vi "Smart Mech Drive.vi"(4 "navX Device":T7={"Interface"={"Protocol"=enum."SPI", "Update Rate (4Hz-100Hz)"=50, "navX Open TypeDef"=variant(cluster{"SPI Bus":enum16{"SPI On-Board, CS0", "SPI On-Board, CS1", "SPI On-Board, CS2", "SPI On-Board, CS3", "SPI MXP", "Invalid"}, "Clock Rate (Hz)":dbl} {"SPI Bus"=enum."SPI MXP", "Clock Rate (Hz)"=2000000.0})}, "Notify Packet"=refnum, "Loop VI Refnum"=refnum, "Ready to Close Occurrence Refnum"=refnum} {"Interface"."Update Rate (4Hz-100Hz)" min=4 max=60 step=1}, 5 "rotation lock":bool, 6 "align":bool, 7 "set_angle":dbl, 10 "motor values":dbl[](array[numeric])=[0.0, 0.0, 0.0, 0.0], 11 "motor references":T1[](array[typedef])=[{"DeviceStatus"={"status"=FALSE, "code"=0, "source"=""}, "Type"=enum."CAN", "PWM"={"PWM Channel"=enum."PWM 1", "DeadBand"={"Name"="", "maxPositivePwm"=0, "minPositivePwm"=0, "centerPwm"=0, "maxNegativePwm"=0, "minNegativePwm"=0, "angularRange"=0}}, "CAN"={"Device Number"=2, "SetOutput VI Ref"=variant(refnum<vi> refnum), "GetOutput VI Ref"=variant(refnum<vi> refnum), "Enable VI Ref"=variant(refnum<vi> refnum), "Disable VI Ref"=variant(refnum<vi> refnum), "Data"=variant(cluster{"Library":path, "handle":u64, "Control Mode":u16, "UsageFrame":u32, "RefNumName":string, "arbID":u32} {"Library"=path "libCTRE_PhoenixCCI.so", "handle"=3032512360, "Control Mode"=0, "UsageFrame"=0, "RefNumName"="drive_fl", "arbID"=33816578})}, "Invert"=TRUE, "DIO PWM"={"PWM \"Enable\" Channel"=enum."Invalid", "DIOChannel"=enum."Invalid", "PWM Rate"=0.0}}, {"DeviceStatus"={"status"=FALSE, "code"=0, "source"=""}, "Type"=enum."CAN", "PWM"={"PWM Channel"=enum."PWM 1", "DeadBand"={"Name"="", "maxPositivePwm"=0, "minPositivePwm"=0, "centerPwm"=0, "maxNegativePwm"=0, "minNegativePwm"=0, "angularRange"=0}}, "CAN"={"Device Number"=4, "SetOutput VI Ref"=variant(refnum<vi> refnum), "GetOutput VI Ref"=variant(refnum<vi> refnum), "Enable VI Ref"=variant(refnum<vi> refnum), "Disable VI Ref"=variant(refnum<vi> refnum), "Data"=variant(cluster{"Library":path, "handle":u64, "Control Mode":u16, "UsageFrame":u32, "RefNumName":string, "arbID":u32} {"Library"=path "libCTRE_PhoenixCCI.so", "handle"=2990105016, "Control Mode"=0, "UsageFrame"=0, "RefNumName"="drive_fr", "arbID"=33816580})}, "Invert"=TRUE, "DIO PWM"={"PWM \"Enable\" Channel"=enum."Invalid", "DIOChannel"=enum."Invalid", "PWM Rate"=0.0}}, {"DeviceStatus"={"status"=FALSE, "code"=0, "source"=""}, "Type"=enum."CAN", "PWM"={"PWM Channel"=enum."PWM 1", "DeadBand"={"Name"="", "maxPositivePwm"=0, "minPositivePwm"=0, "centerPwm"=0, "maxNegativePwm"=0, "minNegativePwm"=0, "angularRange"=0}}, "CAN"={"Device Number"=3, "SetOutput VI Ref"=variant(refnum<vi> refnum), "GetOutput VI Ref"=variant(refnum<vi> refnum), "Enable VI Ref"=variant(refnum<vi> refnum), "Disable VI Ref"=variant(refnum<vi> refnum), "Data"=variant(cluster{"Library":path, "handle":u64, "Control Mode":u16, "UsageFrame":u32, "RefNumName":string, "arbID":u32} {"Library"=path "libCTRE_PhoenixCCI.so", "handle"=3032511496, "Control Mode"=0, "UsageFrame"=0, "RefNumName"="drive_rl", "arbID"=33816579})}, "Invert"=TRUE, "DIO PWM"={"PWM \"Enable\" Channel"=enum."Invalid", "DIOChannel"=enum."Invalid", "PWM Rate"=0.0}}, {"DeviceStatus"={"status"=FALSE, "code"=0, "source"=""}, "Type"=enum."CAN", "PWM"={"PWM Channel"=enum."PWM 1", "DeadBand"={"Name"="", "maxPositivePwm"=0, "minPositivePwm"=0, "centerPwm"=0, "maxNegativePwm"=0, "minNegativePwm"=0, "angularRange"=0}}, "CAN"={"Device Number"=1, "SetOutput VI Ref"=variant(refnum<vi> refnum), "GetOutput VI Ref"=variant(refnum<vi> refnum), "Enable VI Ref"=variant(refnum<vi> refnum), "Disable VI Ref"=variant(refnum<vi> refnum), "Data"=variant(cluster{"Library":path, "handle":u64, "Control Mode":u16, "UsageFrame":u32, "RefNumName":string, "arbID":u32} {"Library"=path "libCTRE_PhoenixCCI.so", "handle"=3006273360, "Control Mode"=0, "UsageFrame"=0, "RefNumName"="drive_rr", "arbID"=33816577})}, "Invert"=FALSE, "DIO PWM"={"PWM \"Enable\" Channel"=enum."Invalid", "DIOChannel"=enum."Invalid", "PWM Rate"=0.0}}]) -> (2 "new motor values":dbl[](array[numeric]), 3 "motor references":T1[](array[typedef]))   [LabVIEW 2018]
uses:
  FIRST-3958-Controls-Library/NavX/navX Library v2/TypeDefs/Z900_navX_DeviceTypeDef.ctl
  FIRST-3958-Controls-Library/NavX/navX Library v2/TypeDefs/Z900_navX_ProtocolTypeDef.ctl
  FIRST-3958-Controls-Library/NavX/navX Library v2/TypeDefs/Z900_navX_NotifyPacketTypeDef.ctl
  FIRST-3958-Controls-Library/NavX/navX Library v2/TypeDefs/Z900_navX_ActionTypeDef.ctl
  <vilib>/Rock Robotics/WPI/MotorControl/WPI_MotorControlDeviceRef.ctl
  <vilib>/Rock Robotics/WPI/MotorControl/WPI_MotorControlType.ctl
  <vilib>/Rock Robotics/SystemInterfaces/DIO/FPGA_DIOPWMChannel.ctl
  <vilib>/Rock Robotics/WPI/PWM/WPI_PWMDeadband.ctl
  <vilib>/Rock Robotics/SystemInterfaces/DIO/FPGA_DIOChannel.ctl
  <vilib>/addons/control/pid/pid.llb/PID (DBL).vi
  Robot Global Data.vi
  <vilib>/addons/control/pid/NI_PID_pid.lvlib
  FIRST-3958-Controls-Library/NavX/navX Library v2/navX Library v2.lvlib
panel:
  in  "PID gains far":T6={"proportional gain (Kc)"=1.0, "integral time (Ti, min)"=0.01, "derivative time (Td, min)"=0.0} {"derivative time (Td, min)" format="%.3f"; "integral time (Ti, min)" format="%.3f"; "proportional gain (Kc)" format="%.3f"}
  in  "PID gains":T6={"proportional gain (Kc)"=1.0, "integral time (Ti, min)"=0.01, "derivative time (Td, min)"=0.0} {"derivative time (Td, min)" format="%.3f"; "integral time (Ti, min)" format="%.3f"; "proportional gain (Kc)" format="%.3f"}
  out "Distance (ft)":dbl=nan
  in  "threshold":dbl
  in  "P":dbl=1.4
  in  "Angle PID":T6={"proportional gain (Kc)"=5.0, "integral time (Ti, min)"=0.0, "derivative time (Td, min)"=0.0} {"derivative time (Td, min)" format="%.3f"; "integral time (Ti, min)" format="%.3f"; "proportional gain (Kc)" format="%.3f"}
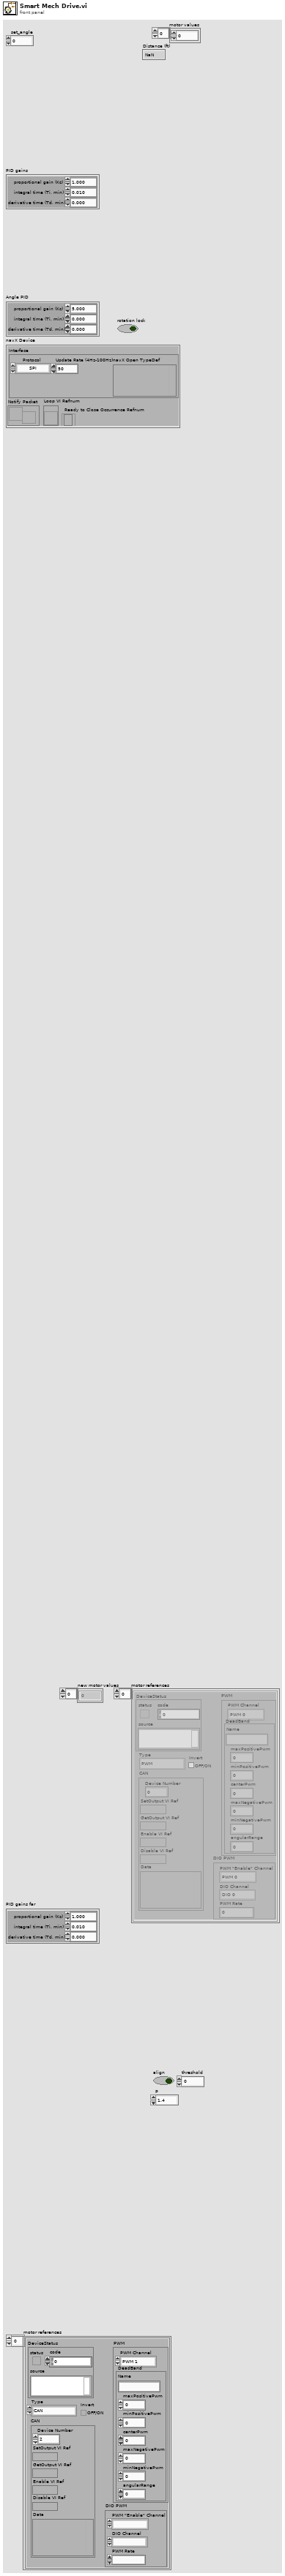
[diagram p1: front panel]
types:
  T1 = typedef "WPI_MotorControlDeviceRef.ctl" = cluster{"DeviceStatus":errorcluster, "Type":T2, "PWM":cluster{"PWM Channel":T3, "DeadBand":T4}, "CAN":cluster{"Device Number":u8, "SetOutput VI Ref":variant, "GetOutput VI Ref":variant, "Enable VI Ref":variant, "Disable VI Ref":variant, "Data":variant}, "Invert":bool, "DIO PWM":cluster{"PWM \"Enable\" Channel":T3, "DIOChannel":T5, "PWM Rate":dbl}}
  T2 = typedef "WPI_MotorControlType.ctl" = enum16{"PWM", "CAN", "DIO PWM"}
  T3 = typedef "FPGA_DIOPWMChannel.ctl" = enum8{"PWM 0", "PWM 1", "PWM 2", "PWM 3", "PWM 4", "PWM 5", "PWM 6", "PWM 7", "PWM 8", "PWM 9", "PWM MXP 0", "PWM MXP 1", "PWM MXP 2", "PWM MXP 3", "PWM MXP 4", "PWM MXP 5", "PWM MXP 6", "PWM MXP 7", "PWM MXP 8", "PWM MXP 9", "Invalid"}
  T4 = typedef "WPI_PWMDeadband.ctl" = cluster{"Name":string, "maxPositivePwm":i32, "minPositivePwm":i32, "centerPwm":i32, "maxNegativePwm":i32, "minNegativePwm":i32, "angularRange":u16}
  T5 = typedef "FPGA_DIOChannel.ctl" = enum8{"DIO 0", "DIO 1", "DIO 2", "DIO 3", "DIO 4", "DIO 5", "DIO 6", "DIO 7", "DIO 8", "DIO 9", "DIO MXP 0", "DIO MXP 1", "DIO MXP 2", "DIO MXP 3", "DIO MXP 4", "DIO MXP 5", "DIO MXP 6", "DIO MXP 7", "DIO MXP 8", "DIO MXP 9", "DIO MXP 10", "DIO MXP 11", "DIO MXP 12", "DIO MXP 13", "DIO MXP 14", "DIO MXP 15", "SPI Port CS1", "SPI Port CS2", "SPI Port CS3", "SPI Port MISO", "SPI Port MOSI", "Invalid"}
  T6 = cluster{"proportional gain (Kc)":dbl, "integral time (Ti, min)":dbl, "derivative time (Td, min)":dbl}
  T7 = typedef "navX Library v2.lvlib/Z900_navX_DeviceTypeDef.ctl" = cluster{"Interface":cluster{"Protocol":T8, "Update Rate (4Hz-100Hz)":u8, "navX Open TypeDef":variant}, "Notify Packet":refnum<notifier>, "Loop VI Refnum":refnum<vi>, "Ready to Close Occurrence Refnum":refnum<k4>}
  T8 = typedef "navX Library v2.lvlib/Z900_navX_ProtocolTypeDef.ctl" = enum16{"SERIAL", "I2C", "SPI"}
  T9 = cluster{"Yaw":dbl, "Roll":dbl, "Pitch":dbl, "Heading":dbl, "Fused Heading":dbl}
  T10 = cluster{"Distance (ft)":dbl, "Score":dbl, "Normalized":cluster{"Center":cluster{dbl, dbl}, "Rectangle":cluster{"Numeric":dbl, "Numeric 2":dbl, "Numeric 3":dbl, "Numeric 5":dbl}}, "Pixels":cluster{"Center":cluster{dbl, dbl}, "Rectangle":cluster{"Numeric":dbl, "Numeric 2":dbl, "Numeric 3":dbl, "Numeric 5":dbl}}}
  T11 = cluster{"Center":cluster{dbl, dbl}, "Rectangle":cluster{"Numeric":dbl, "Numeric 2":dbl, "Numeric 3":dbl, "Numeric 5":dbl}}
  T12 = cluster{"Numeric":dbl, "Numeric 2":dbl, "Numeric 3":dbl, "Numeric 5":dbl}
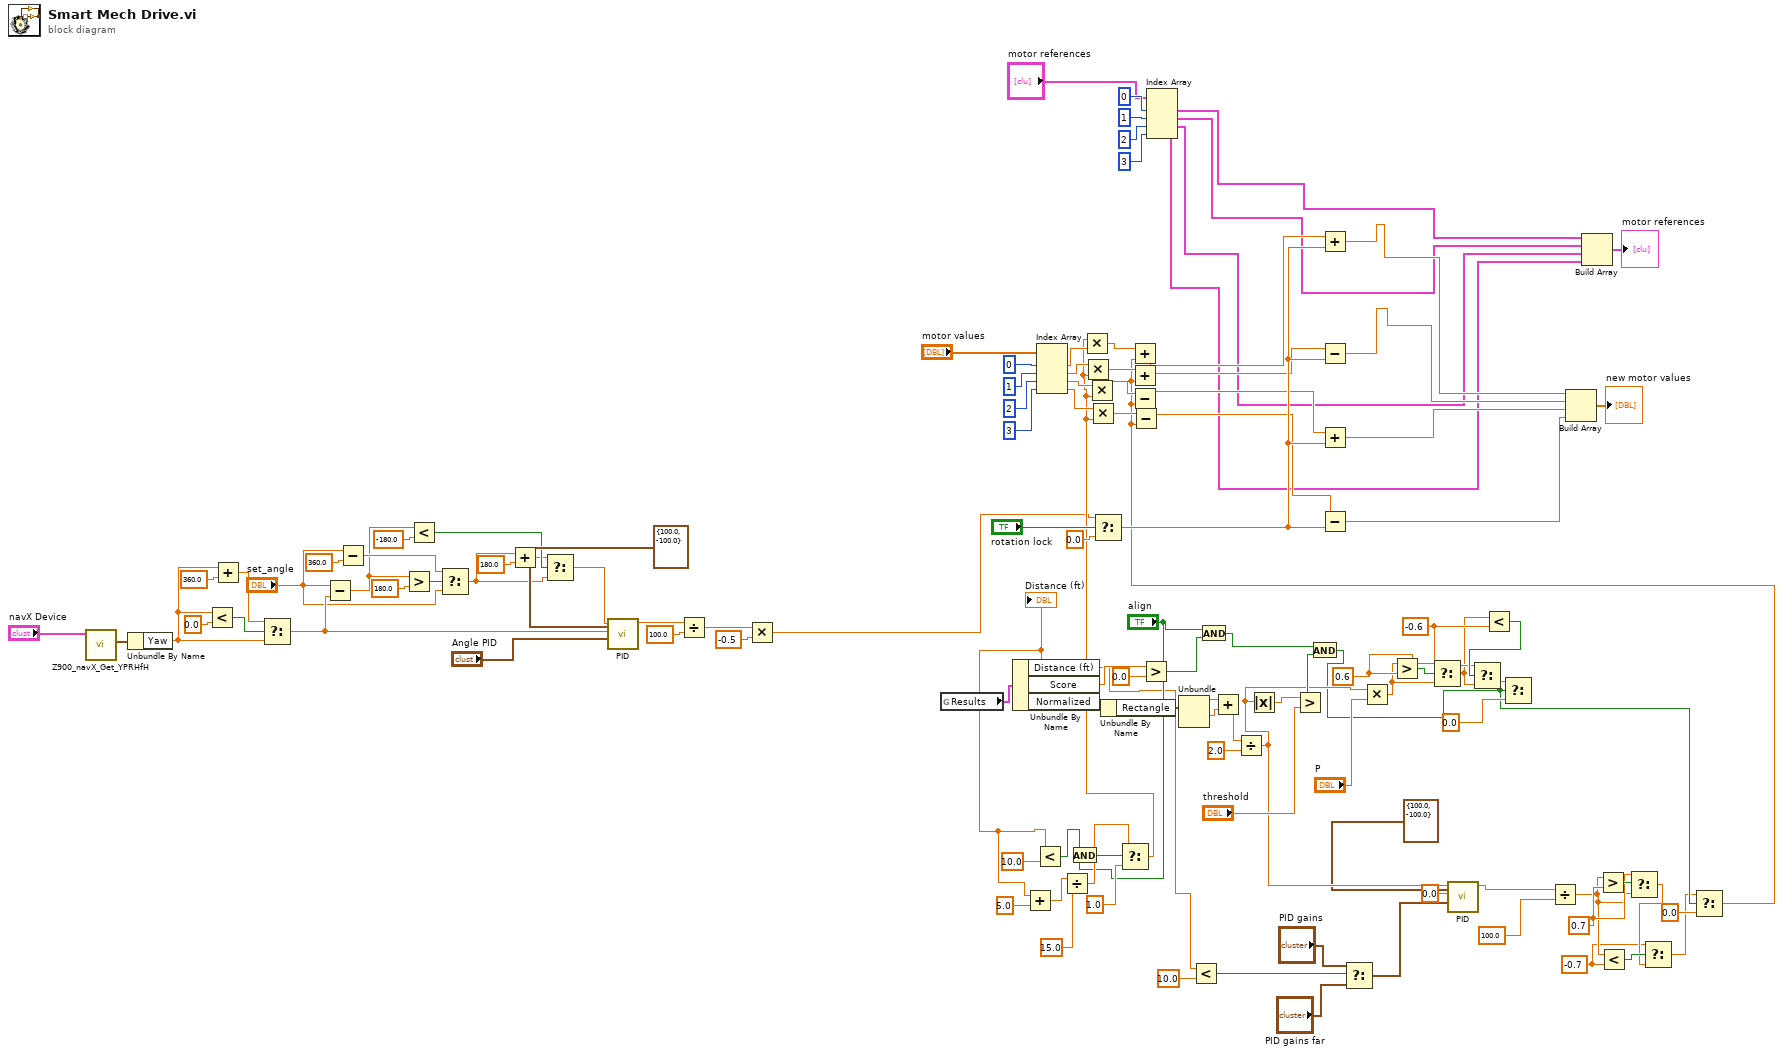
[diagram p0: block diagram]
diagram:
  w30 = -0.7 ("y")
  w34 = 0.7 ("y")
  w82 = -0.6 ("y")
  w84 = 0.6 ("y")
  n1 = call "Z900_navX_Get_YPRHfH.vi"("navX Device"="navX Device") -> ("YRPHfH"=w58:T9)  [unwired: 7 in, 3 out]
  n2 = Unbundle By Name(w58) -> ("Yaw"=w14:dbl)
  n3 = Less?(x=w14, y=0.0) -> (x < y?=w17:bool)
  n4 = Add(x=w14, y=360.0) -> (x+y=w15:dbl)
  n5 = Select(t=w15, s=w17, f=w14) -> (s? t:f=w13:dbl)
  n6 = Subtract(x="set_angle", y=w13) -> (x-y=w6:dbl)
  n7 = Subtract(x="set_angle", y=360.0) -> (x-y=w10:dbl)
  n8 = Greater?(x=w6, y=180.0) -> (0:w11:bool)
  n9 = Less?(x=w6, y=-180.0) -> (x < y?=w5:bool)
  n10 = Select(t=w10, s=w11, f="set_angle") -> (s? t:f=w4:dbl)
  n11 = Add(x=w4, y=180.0) -> (x+y=w3:dbl)
  n12 = Select(t=w3, s=w5, f=w4) -> (s? t:f=w1:dbl)
  n13 = call-poly <vilib>:"PID.vi"("output range"=cluster{"output high":dbl, "output low":dbl} {"output high"=100.0, "output low"=-100.0}, "PID gains"="Angle PID", "process variable"=w13, "setpoint"=w1) -> ("output"=w55:dbl)  [unwired: 6 in, 1 out]
  n14 = Divide(x=w55, y=100.0) -> (x/y=w53:dbl)
  n15 = Multiply(x=w53, y=-0.5) -> (x*y=w51:dbl)
  n16 = global read "Robot Global Data.vi" "Results"() -> (w105:T10)
  n17 = Unbundle By Name(w105) -> ("Distance (ft)"=w38:dbl, "Score"=w103:dbl, "Normalized"=w104:T11)
  "Distance (ft)" <- w38
  n18 = Add(x=w38, y=5.0) -> (x+y=w69:dbl)
  n19 = Less?(x=w38, y=10.0) -> (x < y?=w71:bool)
  n20 = Index Array(array="motor values", index #1=0 ("index"), index #2=1 ("index"), index #3=2 ("index"), index #4=3 ("index")) -> (element #1=w94:dbl, element #2=w108:dbl, element #3=w107:dbl, element #4=w106:dbl)
  n21 = Divide(x=w69, y=15.0) -> (x/y=w66:dbl)
  n22 = And(x=w71, y="align") -> (x .and. y?=w65:bool)
  n23 = Select(t=w51, s="rotation lock", f=0.0) -> (s? t:f=w110:dbl)
  n24 = Unbundle By Name(w104) -> ("Rectangle"=w89:T12)
  n25 = Select(t=w66, s=w65, f=1.0 ("t")) -> (s? t:f=w59:dbl)
  n26 = Multiply(x=w59, y=w94) -> (x*y=w63:dbl)
  n27 = Multiply(x=w108, y=w59) -> (x*y=w62:dbl)
  n28 = Multiply(x=w107, y=w59) -> (x*y=w61:dbl)
  n29 = Multiply(x=w106, y=w59) -> (x*y=w60:dbl)
  n30 = Greater?(x=w103, y=0.0) -> (0:w101:bool)
  n31 = Index Array(array="motor references", index #1=0 ("index"), index #2=1 ("index"), index #3=2 ("index"), index #4=3 ("index")) -> (element #1=w22:T1, element #2=w21:T1, element #3=w20:T1, element #4=w19:T1)
  n32 = Unbundle(w89) -> ("Numeric"=w88:dbl, "Numeric 3"=w78:dbl)  [unwired: 2 out]
  n33 = Less?(x=w38, y=10.0) -> (x < y?=w36:bool)
  n34 = And(x="align", y=w101) -> (x .and. y?=w99:bool)
  n35 = Add(x=w88, y=w78) -> (x+y=w87:dbl)
  n36 = Divide(x=w87, y=2.0) -> (x/y=w49:dbl)
  n37 = Absolute Value(x=w49) -> (abs(x)=w100:dbl)
  n38 = Greater?(x=w100, y="threshold") -> (0:w98:bool)
  n39 = And(x=w99, y=w98) -> (x .and. y?=w43:bool)
  n40 = Select(t="PID gains", s=w36, f="PID gains far") -> (s? t:f=w39:T6)
  n41 = Multiply(x=w49, y="P") -> (x*y=w80:dbl)
  n42 = Greater?(x=w80, y=w84) -> (0:w85:bool)
  n43 = Select(t=w84, s=w85, f=w80) -> (s? t:f=w81:dbl)
  n44 = call-poly <vilib>:"PID.vi"("output range"=cluster{"output high":dbl, "output low":dbl} {"output high"=100.0, "output low"=-100.0}, "PID gains"=w39, "process variable"=0.0, "setpoint"=w49) -> ("output"=w46:dbl)  [unwired: 6 in, 1 out]
  n45 = Less?(x=w81, y=w82) -> (x < y?=w83:bool)
  n46 = Select(t=w82, s=w83, f=w81) -> (s? t:f=w79:dbl)
  n47 = Select(t=w79, s=w43, f=0.0 ("t")) -> ()  [unwired: 1 out]
  n48 = Divide(x=w46, y=100.0) -> (x/y=w33:dbl)
  n49 = Build Array(w22, w21, w20, w19) -> (→"motor references":T1[])
  n50 = Greater?(x=w33, y=w34) -> (0:w35:bool)
  n51 = Less?(x=w33, y=w30) -> (x < y?=w32:bool)
  n52 = Select(t=w34, s=w35, f=w33) -> (s? t:f=w31:dbl)
  n53 = Select(t=w30, s=w32, f=w31) -> (s? t:f=w29:dbl)
  n54 = Select(t=w29, s=w43, f=0.0) -> (s? t:f=w42:dbl)
  n55 = Add(x=w63, y=w42) -> (x+y=w95:dbl)
  n56 = Add(x=w62, y=w42) -> (x+y=w93:dbl)
  n57 = Subtract(x=w61, y=w42) -> (x-y=w92:dbl)
  n58 = Subtract(x=w60, y=w42) -> (x-y=w91:dbl)
  n59 = Add(x=w95, y=w110) -> (x+y=w27:dbl)
  n60 = Subtract(x=w93, y=w110) -> (x-y=w26:dbl)
  n61 = Add(x=w92, y=w110) -> (x+y=w25:dbl)
  n62 = Subtract(x=w91, y=w110) -> (x-y=w24:dbl)
  n63 = Build Array(w27, w26, w25, w24) -> (→"new motor values":dbl[])
